vi "camara 2.1.vi"() -> ()   [LabVIEW 2010]
uses:
  <vilib>/addons/PixeLINK/Low Level Functions/CAMERA_FEATURES.llb/TDPU-CameraFeatures-FeatureIds.ctl
  <vilib>/addons/PixeLINK/Low Level Functions/CAMERA_FEATURES.llb/TDPU-CameraFeatures-FeatureFlags.ctl
  <vilib>/addons/PixeLINK/Low Level Functions/ACQUISITION.llb/TDPU-Acquisition-StreamState.ctl
  <vilib>/sound2/lvsound2.llb/Sampling Mode.ctl
  <vilib>/vision/NI_Vision_Development_Module.lvlib
  <vilib>/addons/PixeLINK/Low Level Functions/CAMERA_FEATURES.llb/TDPU-CameraFeatures-PixelFormat.ctl
  <vilib>/sound2/lvsound2.llb/Sound Data Format.ctl
panel:
  in  "SigmaMax (ms)":dbl
  in  "lamda (nm)":dbl
  in  "m":dbl
  in  "b":dbl
  in  "opticalPathMax (nm)":dbl
  out "contraste":u8
  in  "Sonido":bool
  in  "lamda (nm)":dbl
  in  "Frecuencia":dbl
  in  "sound format":T1={"sample rate (S/s)"=22050.0, "number of channels"=2, "bits per sample"=16}
  in  "Mostrar":bool
  in  "Blue":sgl(slide) scale=0.0..4.0
  in  "Green":sgl(slide) scale=0.0..4.0
  in  "Red":sgl(slide) scale=0.0..4.0
  in  "Gain":dbl(slide) scale=0.0..25.0
  out "Image":T2(plugin-control)
  in  "Exposure Time (ms)":dbl(slide) scale=0.1..2000.0
  in  "Streeam":bool
  in  "Pixel Format Requerido":T3 items=["PIXEL_FORMAT_MONO8", "PIXEL_FORMAT_MONO16", "PIXEL_FORMAT_YUV422", "PIXEL_FORMAT_BAYER8_GRBG", "PIXEL_FORMAT_BAYER16_GRBG", "PIXEL_FORMAT_RGB24", "PIXEL_FORMAT_RGB48", "PIXEL_FORMAT_BAYER8_RGGB", "PIXEL_FORMAT_BAYER8_GBRG ", "PIXEL_FORMAT_BAYER8_BGGR ", "PIXEL_FORMAT_BAYER16_RGGB ", "PIXEL_FORMAT_BAYER16_GBRG", "PIXEL_FORMAT_BAYER16_BGGR", "PIXEL_FORMAT_RGB32"]
  in  "Stop App":bool
  out "Numero de Camaras":u32
  in  "Selector":u16(ring) items=["776002034"]
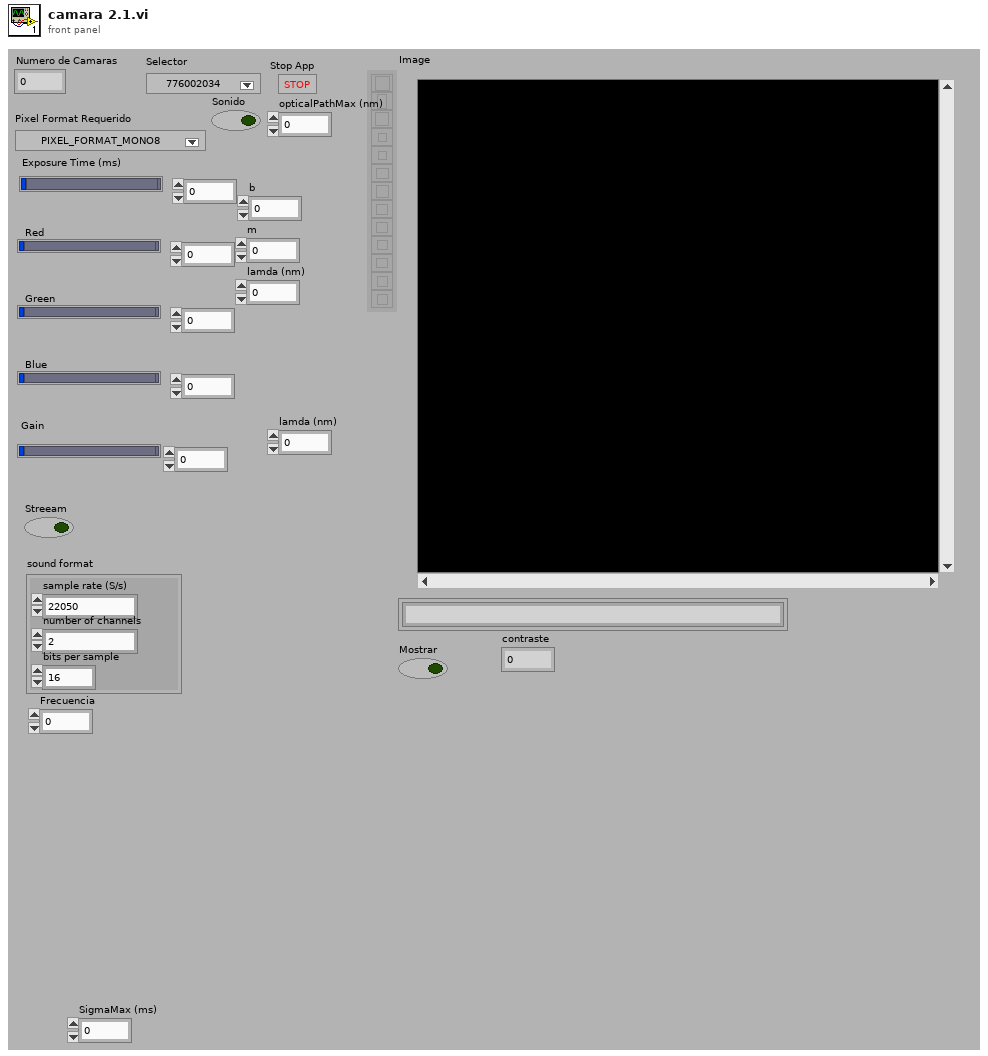
[diagram p1: front panel]
types:
  T1 = typedef "Sound Data Format.ctl" = cluster{"sample rate (S/s)":dbl, "number of channels":i32, "bits per sample":i32}
  T2 = typedef "IMAQ Image.ctl" = refnum<image>
  T3 = typedef "TDPU-CameraFeatures-PixelFormat.ctl" = u16
  T4 = typedef "Sampling Mode.ctl" = i32
  T5 = typedef "Image Type" = u32
  T6 = cluster{"sample rate (S/s)":dbl, "number of channels":i32, "bits per sample":i32}
  T7 = typedef "Sound Output Task ID.ctl" = u32
  T8 = cluster{"Red (or Hue) value":u8, "Green (or Sat) value":u8, "Blue (or Light or Val) value":u8}[]
  T9 = typedef "TDPU-Acquisition-StreamState.ctl" = u32
  T10 = typedef "TDPU-CameraFeatures-FeatureIds.ctl" = u32
  T11 = typedef "TDPU-CameraFeatures-FeatureFlags.ctl" = u32
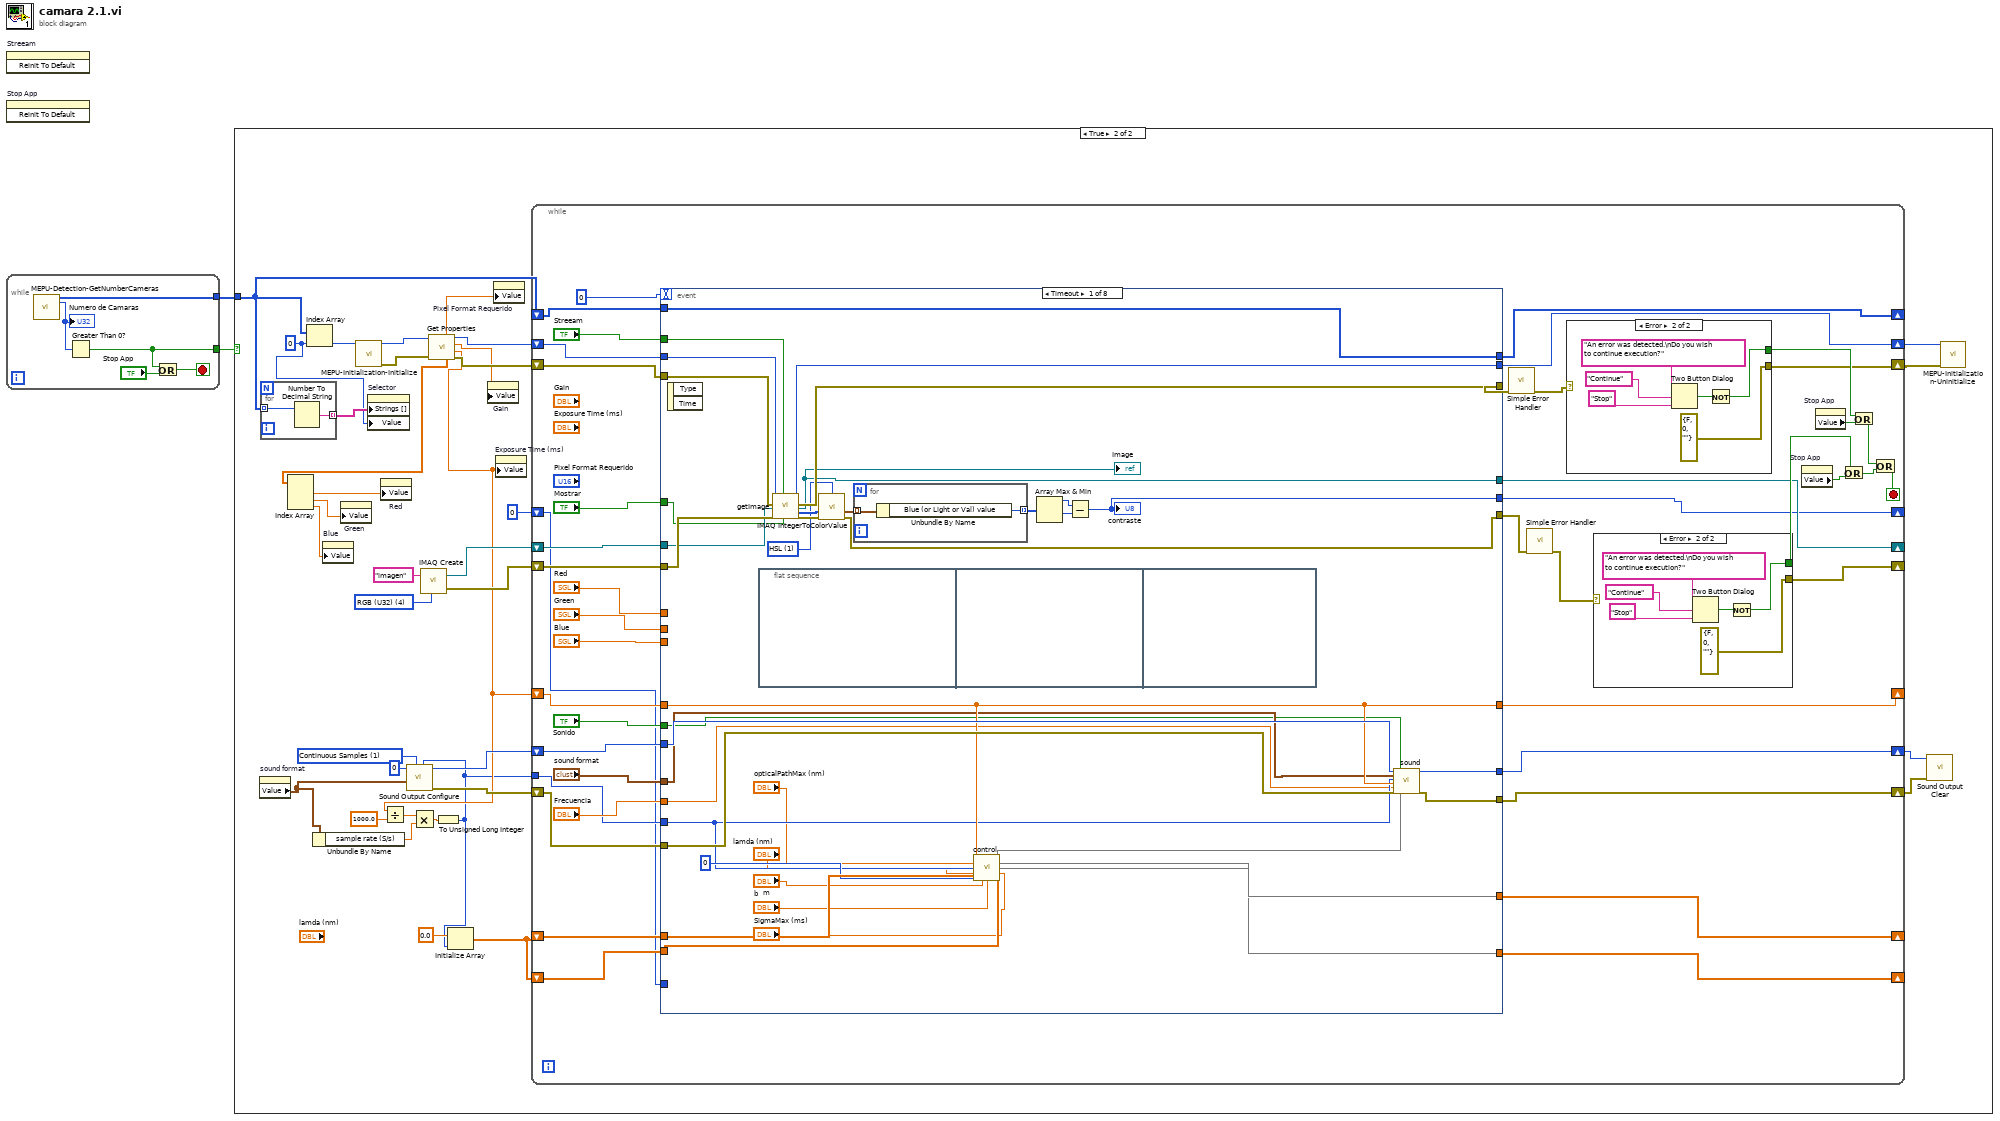
[diagram p0: block diagram]
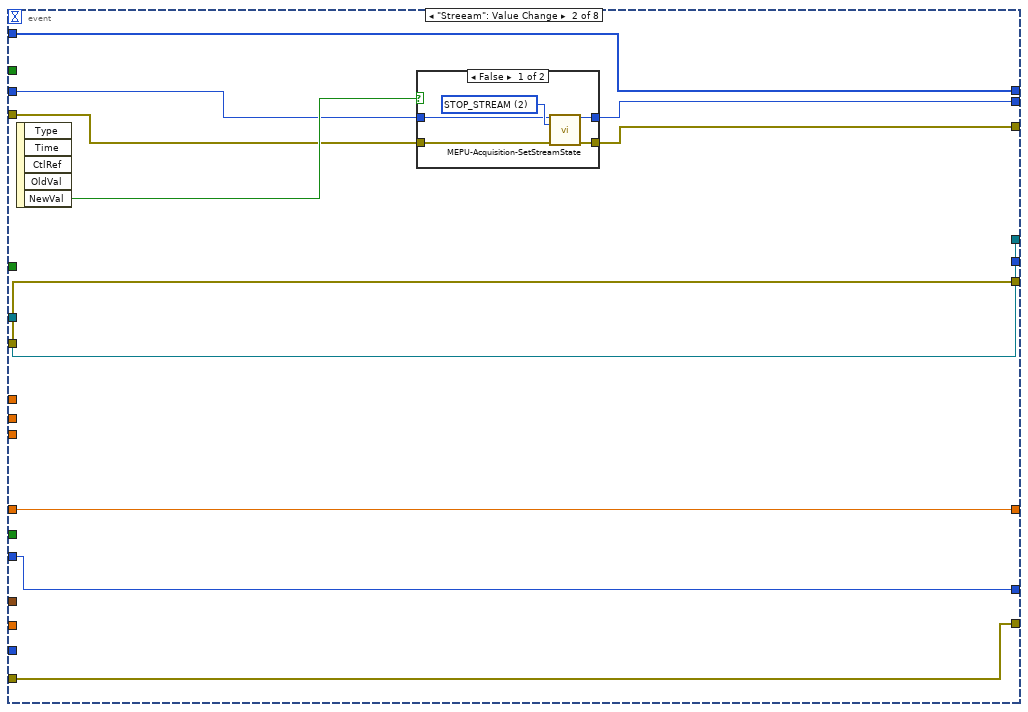
[diagram p5: hidden frame]
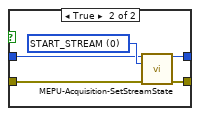
[diagram p6: hidden frame]
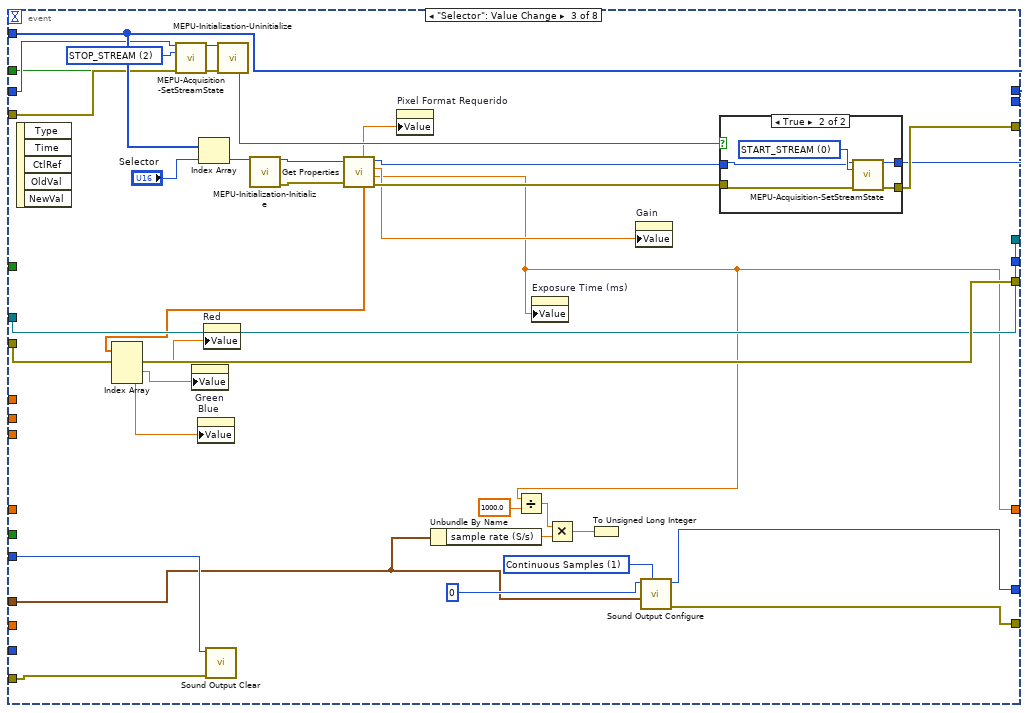
[diagram p7: hidden frame]
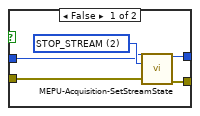
[diagram p8: hidden frame]
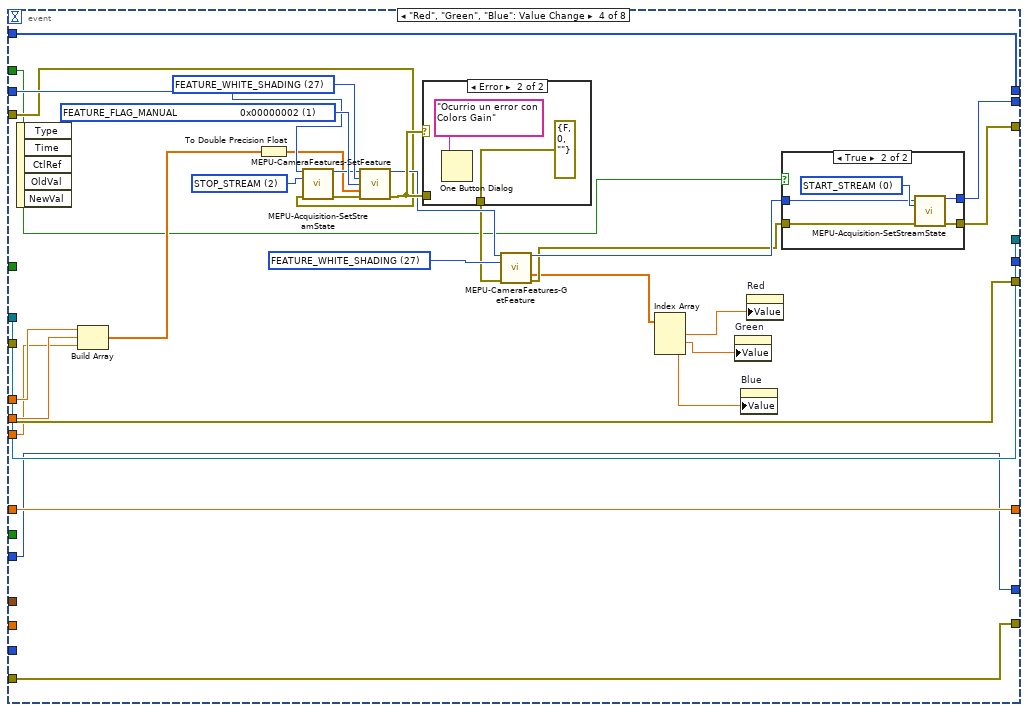
[diagram p9: hidden frame]
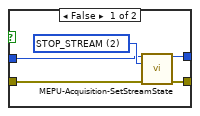
[diagram p10: hidden frame]
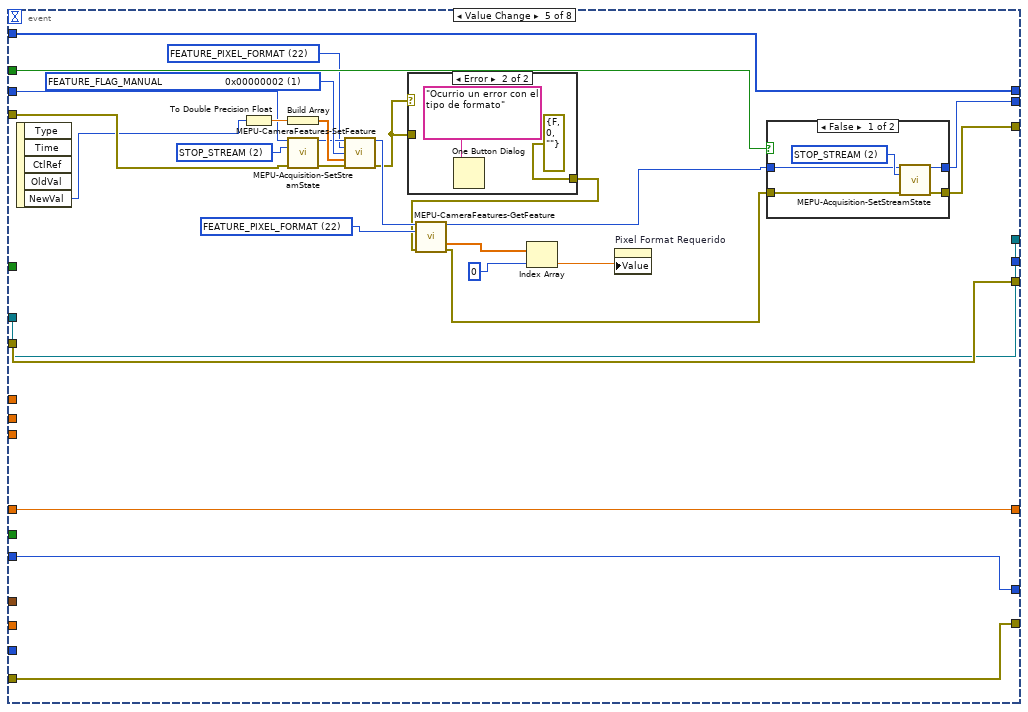
[diagram p12: hidden frame]
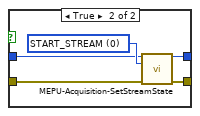
[diagram p13: hidden frame]
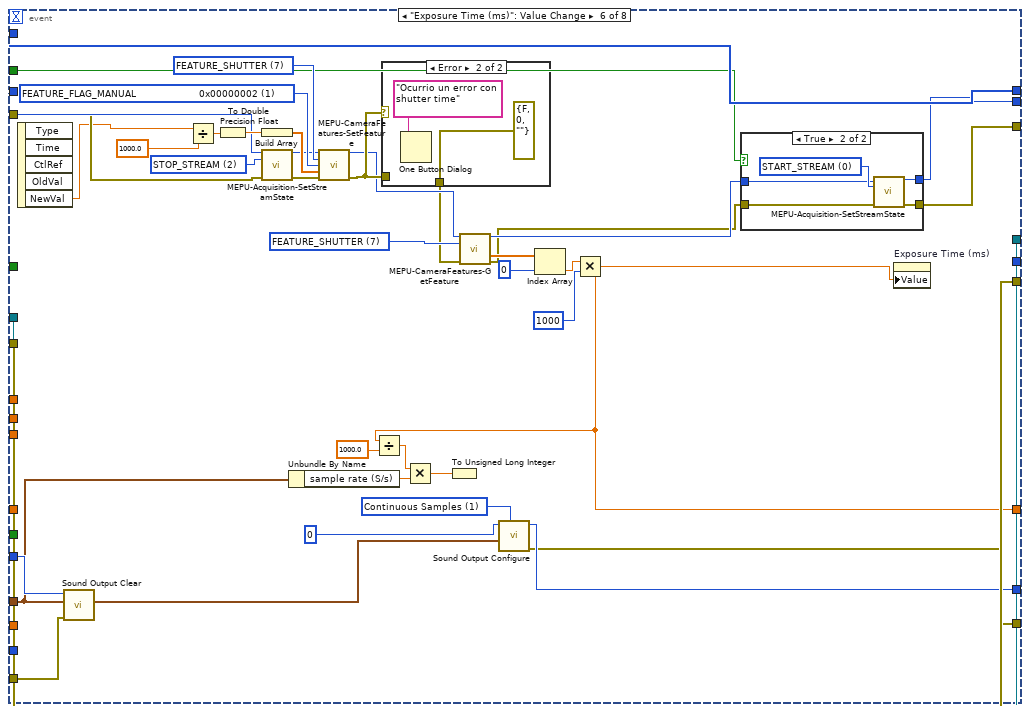
[diagram p15: hidden frame]
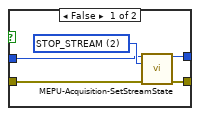
[diagram p16: hidden frame]
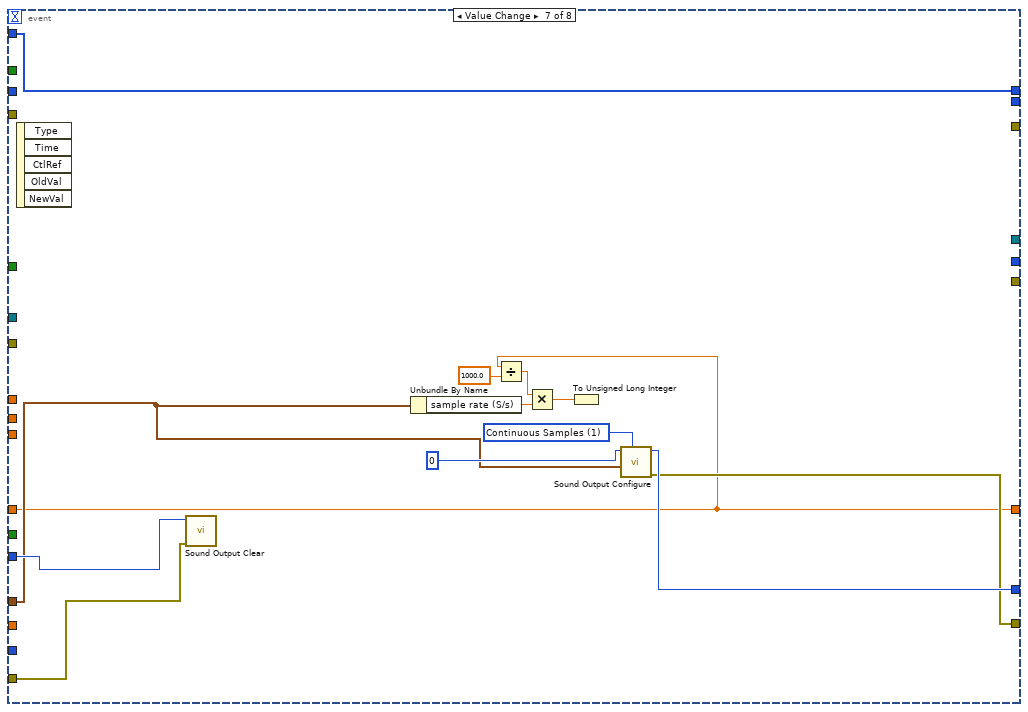
[diagram p18: hidden frame]
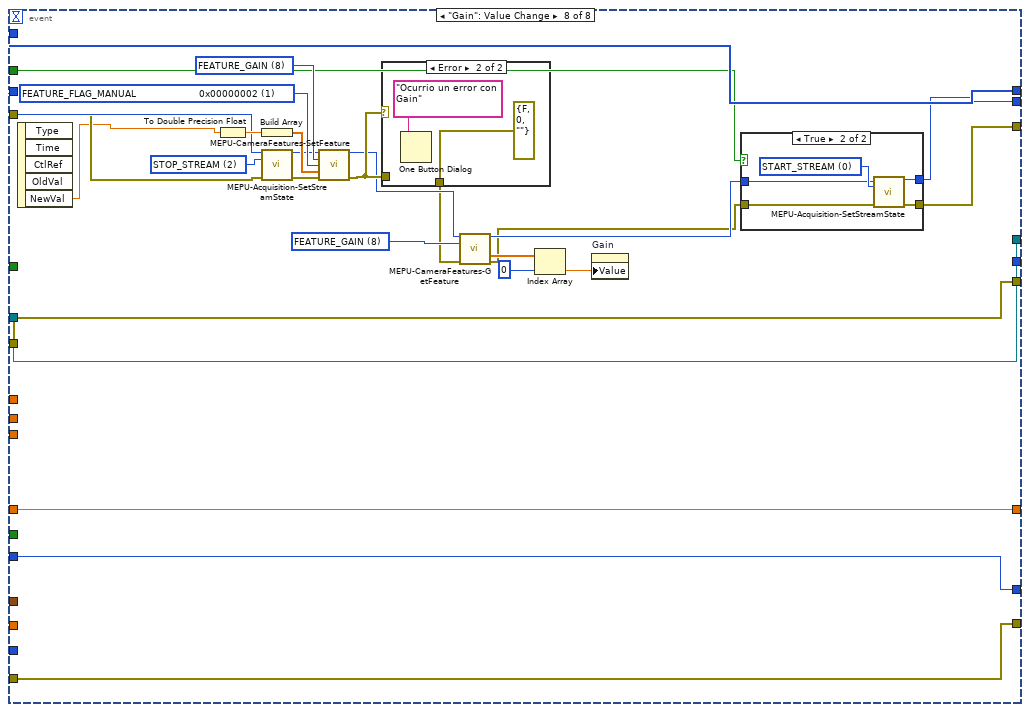
[diagram p19: hidden frame]
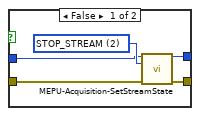
[diagram p20: hidden frame]
diagram:
  n1 = invoke on="Streeam" class="Bool (strict)" method="Reinit To Default"() -> ()  [unwired: 3 in, 3 out]
  n2 = invoke on="Stop App" class="Bool (strict)" method="Reinit To Default"() -> ()  [unwired: 3 in, 3 out]
  n3 = while {
    tunnel: [w7] -> w2
    tunnel: [w3] -> w1
    stop <- w5 stop-if-true
    n4 = call <vilib>:"MEPU-Detection-GetNumberCameras.vi"() -> ("LV_SerialNumbers OUT"=w7:u32[], "LV_NumberSerial OUT"=w4:u32)  [unwired: 13 in, 1 out]
    "Numero de Camaras" <- w4
    n5 = Greater Than 0?(x=w4) -> (x > 0?=w3:bool)
    n6 = Or(x=w3, y="Stop App") -> (x .or. y?=w5:bool)
  }
  n7 = case shown="True" w1 {
    tunnel: w2 -> [_ w41]
    frame False {
    }
    frame True {
      w24 = T4 1 items=["Finite Samples", "Continuous Samples"] ("sample mode")
      w35 = T5 4 items=["Grayscale (U8)", "Grayscale (I16)", "Grayscale (SGL)", "Complex (CSG)", "RGB (U32)", "HSL (U32)", "RGB (U64)", "Grayscale (U16)"] ("Image Type")
      w40 = 0
      n8 = property on="sound format" class="Clust (strict)"() -> ("Value"=w16:T6)  [unwired: 2 in, 2 out]
      n9 = for {
        tunnel: w41 -> [w403] mode=indexing
        tunnel: [w402] -> w43 mode=indexing
        n10 = Number To Decimal String(number=w403) -> (decimal integer string=w402:string)  [unwired: 1 in]
      }
      n11 = Index Array(array=w41, index=w40) -> (element=w42:u32)
      n12 = Unbundle By Name(w16) -> ("sample rate (S/s)"=w20:dbl)
      n13 = call <vilib>:"MEPU-Initialization-Initialize.vi"("uSerialNumber IN"=w42) -> ("phCamera OUT"=w34:u32, "Error OUT"=w33:errorcluster)  [unwired: 12 in, 1 out]
      n14 = property on="Selector" class="Ring (strict)"("Strings []"=w43, "Value"=w40) -> ()  [unwired: 2 in, 2 out]
      n15 = call "IMAQ Create"("Image Name"="imagen", "Image Type"=w35) -> ("New Image"=w38:T2, "error out"=w36:errorcluster)  [unwired: 3 in]
      n16 = call "Get Properties.vi"("hCamera IN"=w34, "Error IN"=w33) -> ("Pixel Format OUT"=w30:dbl, "hCamera OUT"=w32:u32, "Gain OUT"=w29:dbl, "Colors Gain OUT"=w25:dbl[], "Shutter Time OUT (ms)"=w15:dbl, "Error OUT"=w31:errorcluster)  [unwired: 3 in]
      n17 = Index Array(array=w25) -> (element #1=w28:dbl, element #2=w27:dbl, element #3=w26:dbl)  [unwired: 3 in]
      n18 = property on="Blue" class="Slide (strict)"("Value"=w26) -> ()  [unwired: 2 in, 2 out]
      n19 = property on="Green" class="Slide (strict)"("Value"=w27) -> ()  [unwired: 2 in, 2 out]
      n20 = property on="Red" class="Slide (strict)"("Value"=w28) -> ()  [unwired: 2 in, 2 out]
      n21 = Divide(x=w15, y=sgl 1000.0) -> (x/y=w19:dbl)
      n22 = Multiply(x=w19, y=w20) -> (x*y=w18:dbl)
      n23 = To Unsigned Long Integer(number=w18) -> (unsigned 32bit integer=w10:u32)
      n24 = call <vilib>:"Sound Output Configure.vi"("number of samples/ch"=w10, "sample mode"=w24, "sound format"=w16, "device ID"=u32 0) -> ("error out"=w21:errorcluster, "task ID"=w22:T7)  [unwired: 6 in]
      n25 = Initialize Array(0.0 ("element"), w10) -> (w9:dbl[])
      n26 = property on="Gain" class="Slide (strict)"("Value"=w29) -> ()  [unwired: 2 in, 2 out]
      n27 = property on="Pixel Format Requerido" class="Ring (strict)"("Value"=w30) -> ()  [unwired: 2 in, 2 out]
      n28 = property on="Exposure Time (ms)" class="Slide (strict)"("Value"=w15) -> ()  [unwired: 2 in, 2 out]
      n29 = while {
        shift-right: [w85] -> _
        shift-left: w41 -> [w86]
        shift-right: [w76] -> w39
        shift-left: w32 -> [w84]
        shift-right: [w80] -> w14
        shift-left: w31 -> [w83]
        shift-right: [w66] -> _
        shift-left: w36 -> [w65]
        shift-right: [w64] -> _
        shift-left: w38 -> [w74]
        shift-right: [w56] -> w13
        shift-left: w22 -> [w59]
        shift-right: [w55] -> w12
        shift-left: w21 -> [w58]
        shift-right: [w54] -> _
        shift-left: w15 -> [w53]
        shift-right: [w46] -> _
        shift-left: w9 -> [w50]
        shift-right: [w49] -> _
        shift-left: w9 -> [w48]
        tunnel: w10 -> [w47]
        shift-right: [w45] -> _
        shift-left: u8 0 -> [w44]
        stop <- w68 stop-if-true
        n30 = event shown="[0] Timeout" {
          selector: _ -> [_ _ _ _ _ _ _ _]
          dyn-events: _ -> [_ _ _ _ _ _ _ _]
          timeout: 0 -> [_ _ _ _ _ _ _ _]
          tunnel: w86 -> [w141 w147 w197 w240 w273 w326 w360 w380]
          tunnel: [w138 w151 w190 w224 w272 w325 _ w379] -> w76
          tunnel: [w137 w150 w191 w223 w271 w324 _ w378] -> w77
          tunnel: [w141 w147 w197 w240 w273 w326 w360 w380] -> w85
          tunnel: w84 -> [w140 w153 w192 w226 w278 w323 _ w377]
          tunnel: w83 -> [w139 w152 w193 w225 w277 w322 _ w376]
          tunnel: "Streeam" -> [w134 _ w189 w213 w270 w321 _ w375]
          tunnel: w74 -> [w135 w148 w187 w228 w258 w307 _ w366]
          tunnel: w65 -> [w136 w149 w188 w227 w269 w318 _ w374]
          tunnel: [w128 w149 w188 w227 w269 w318 _ w374] -> w73
          tunnel: [w133 w148 w187 w228 w258 w307 _ w366] -> w64
          tunnel: "Red" -> [_ _ _ w218 _ _ _ _]
          tunnel: "Green" -> [_ _ _ w217 _ _ _ _]
          tunnel: "Blue" -> [_ _ _ w216 _ _ _ _]
          tunnel: "Mostrar" -> [w132 _ _ _ _ _ _ _]
          tunnel: w59 -> [w118 w145 w170 w211 w255 w306 w353 w362]
          tunnel: w58 -> [w119 w144 w169 w210 w254 w305 w352 w361]
          tunnel: "sound format" -> [w114 _ w165 _ _ w298 w351 _]
          tunnel: [w112 w145 w168 w211 w255 w297 w350 w362] -> w56
          tunnel: [w111 w144 w167 w210 w254 w296 w349 w361] -> w55
          tunnel: w53 -> [w117 w146 _ w212 w256 _ w348 w363]
          tunnel: [w117 w146 w166 w212 w256 w295 w348 w363] -> w54
          tunnel: "Frecuencia" -> [w115 _ _ _ _ _ _ _]
          tunnel: "Sonido" -> [w113 _ _ _ _ _ _ _]
          tunnel: w50 -> [w123 _ _ _ _ _ _ _]
          tunnel: [w122 _ _ _ _ _ _ _] -> w49
          tunnel: w48 -> [w121 _ _ _ _ _ _ _]
          tunnel: w47 -> [w116 _ _ _ _ _ _ _]
          tunnel: [w110 _ _ _ _ _ _ _] -> w46
          tunnel: [w108 _ _ _ _ _ _ _] -> w45
          tunnel: w44 -> [_ _ _ _ _ _ _ _]
          event Timeout {
            w129 = u16 1 items=["RGB", "HSL", "HSV", "HSI"] ("Color Mode")
            n31 = event-data() -> ()  [unwired: 1 in, 2 out]
            n32 = flat-sequence {
              frame #0 {
              }
              frame #1 {
              }
              frame #2 {
              }
            }
            n33 = call "getImage.vi"("hCamera IN"=w140, "errorCamera IN"=w139, "Image IN"=w135, "imageError IN"=w136, "Streeam"=w134, "Show"=w132) -> ("hCamera OUT"=w138:u32, "errorCamera OUT"=w137:errorcluster, "Image OUT"=w133:T2, "1D RGB32 Array OUT"=w131:u32[], "errorImage OUT"=w130:errorcluster)  [unwired: 8 in, 1 out]
            "Image" <- w133
            n34 = call "IMAQ IntegerToColorValue"("error in (no error)"=w130, "1D U32 array"=w131, "Color Mode"=w129) -> ("1D Color value array"=w127:T8, "error out"=w128:errorcluster)  [unwired: 2 in, 2 out]
            n35 = for {
              tunnel: w127 -> [w143] mode=indexing
              tunnel: [w142] -> w126 mode=indexing
              n36 = Unbundle By Name(w143) -> ("Blue (or Light or Val) value"=w142:u8)
            }
            n37 = call "control.vi"("tiempo (ms)"=w117, "opticalPathMax (nm)"="opticalPathMax (nm)", "#samples"=w116, "lamda (nm)"="lamda (nm)", "SigmaMax (ms)"="SigmaMax (ms)", 11:0, "m"="m", "b"="b", 14:w121, 15:w123) -> (4:w109, 6:w122, 8:w110)  [unwired: 3 in]
            n38 = Array Max & Min(array=w126) -> (max value=w125:u8, min value=w124:u8)  [unwired: 2 out]
            n39 = Subtract(x=w125, y=w124) -> (x-y=w108:u8)
            "contraste" <- w108
            n40 = call "sound.vi"("task ID IN"=w118, "sound format"=w114, "# samples"=w116, "time (ms)"=w117, "Base frecuency"=w115, "error IN"=w119, "sound?"=w113, "df Array"=w109) -> ("task ID OUT"=w112:T7, "error OUT"=w111:errorcluster)  [unwired: 10 in]
          }
          event "Streeam": Value Change {
            n41 = event-data() -> ("NewVal"=w154:bool)  [unwired: 1 in, 4 out]
            n42 = case shown="False" w154 {
              tunnel: w153 -> [w158 w163]
              tunnel: w152 -> [w157 w162]
              tunnel: [w155 w161] -> w150
              tunnel: [w156 w160] -> w151
              frame False {
                w159 = T9 2 items=["START_STREAM", "PAUSE_STREAM", "STOP_STREAM"] ("uStreamState IN")
                n43 = call <vilib>:"MEPU-Acquisition-SetStreamState.vi"("hCamera IN"=w158, "uStreamState IN"=w159, "Error IN"=w157) -> ("hCamera OUT"=w156:u32, "Error OUT"=w155:errorcluster)  [unwired: 11 in]
              }
              frame True {
                w164 = T9 0 items=["START_STREAM", "PAUSE_STREAM", "STOP_STREAM"] ("uStreamState IN")
                n44 = call <vilib>:"MEPU-Acquisition-SetStreamState.vi"("hCamera IN"=w163, "uStreamState IN"=w164, "Error IN"=w162) -> ("hCamera OUT"=w160:u32, "Error OUT"=w161:errorcluster)  [unwired: 11 in]
              }
            }
          }
          event "Selector": Value Change {
            w176 = T4 1 items=["Finite Samples", "Continuous Samples"] ("sample mode")
            w196 = T9 2 items=["START_STREAM", "PAUSE_STREAM", "STOP_STREAM"] ("uStreamState IN")
            n45 = event-data() -> ()  [unwired: 1 in, 5 out]
            n46 = call <vilib>:"MEPU-Acquisition-SetStreamState.vi"("hCamera IN"=w192, "uStreamState IN"=w196, "Error IN"=w193) -> ("hCamera OUT"=w194:u32, "Error OUT"=w195:errorcluster)  [unwired: 11 in]
            n47 = Index Array(array=w197, index="Selector") -> (element=w198:u32)
            n48 = call <vilib>:"Sound Output Clear.vi"("error in (no error)"=w169, "task ID"=w170) -> ()  [unwired: 9 in, 1 out]
            n49 = call <vilib>:"MEPU-Initialization-Uninitialize.vi"("hCamera IN"=w194, "Error IN"=w195) -> ()  [unwired: 13 in, 1 out]
            n50 = call <vilib>:"MEPU-Initialization-Initialize.vi"("uSerialNumber IN"=w198) -> ("phCamera OUT"=w183:u32, "Error OUT"=w182:errorcluster)  [unwired: 12 in, 1 out]
            n51 = call "Get Properties.vi"("hCamera IN"=w183, "Error IN"=w182) -> ("Pixel Format OUT"=w181:dbl, "hCamera OUT"=w179:u32, "Gain OUT"=w178:dbl, "Colors Gain OUT"=w177:dbl[], "Shutter Time OUT (ms)"=w166:dbl, "Error OUT"=w180:errorcluster)  [unwired: 3 in]
            n52 = Index Array(array=w177) -> (element #1=w186:dbl, element #2=w185:dbl, element #3=w184:dbl)  [unwired: 3 in]
            n53 = property on="Green" class="Slide (strict)"("Value"=w185) -> ()  [unwired: 2 in, 2 out]
            n54 = property on="Blue" class="Slide (strict)"("Value"=w184) -> ()  [unwired: 2 in, 2 out]
            n55 = property on="Red" class="Slide (strict)"("Value"=w186) -> ()  [unwired: 2 in, 2 out]
            n56 = property on="Pixel Format Requerido" class="Ring (strict)"("Value"=w181) -> ()  [unwired: 2 in, 2 out]
            n57 = Unbundle By Name(w165) -> ("sample rate (S/s)"=w174:dbl)
            n58 = Divide(x=w166, y=sgl 1000.0) -> (x/y=w173:dbl)
            n59 = property on="Exposure Time (ms)" class="Slide (strict)"("Value"=w166) -> ()  [unwired: 2 in, 2 out]
            n60 = Multiply(x=w173, y=w174) -> (x*y=w172:dbl)
            n61 = To Unsigned Long Integer(number=w172) -> ()  [unwired: 1 out]
            n62 = property on="Gain" class="Slide (strict)"("Value"=w178) -> ()  [unwired: 2 in, 2 out]
            n63 = call <vilib>:"Sound Output Configure.vi"("sample mode"=w176, "sound format"=w165, "device ID"=u32 0) -> ("error out"=w167:errorcluster, "task ID"=w168:T7)  [unwired: 7 in]
            n64 = case shown="True" w189 {
              tunnel: [w202 w208] -> w191
              tunnel: [w203 w207] -> w190
              tunnel: w180 -> [w201 w206]
              tunnel: w179 -> [w200 w205]
              frame False {
                w204 = T9 2 items=["START_STREAM", "PAUSE_STREAM", "STOP_STREAM"] ("uStreamState IN")
                n65 = call <vilib>:"MEPU-Acquisition-SetStreamState.vi"("hCamera IN"=w200, "uStreamState IN"=w204, "Error IN"=w201) -> ("hCamera OUT"=w203:u32, "Error OUT"=w202:errorcluster)  [unwired: 11 in]
              }
              frame True {
                w209 = T9 0 items=["START_STREAM", "PAUSE_STREAM", "STOP_STREAM"] ("uStreamState IN")
                n66 = call <vilib>:"MEPU-Acquisition-SetStreamState.vi"("hCamera IN"=w205, "uStreamState IN"=w209, "Error IN"=w206) -> ("hCamera OUT"=w207:u32, "Error OUT"=w208:errorcluster)  [unwired: 11 in]
              }
            }
          }
          event "Red", "Green", "Blue": Value Change {
            w233 = T10 27 items=["FEATURE_BRIGHTNESS", "FEATURE_EXPOSURE", "FEATURE_SHARPNESS", "FEATURE_WHITE_BAL", "FEATURE_HUE", "FEATURE_SATURATION", "FEATURE_GAMMA", "FEATURE_SHUTTER", "FEATURE_GAIN", "FEATURE_IRIS", "FEATURE_FOCUS", "FEATURE_TEMPERATURE", "FEATURE_TRIGGER", "FEATURE_ZOOM", "FEATURE_PAN", "FEATURE_TILT", "FEATURE_OPT_FILTER", "FEATURE_GPIO", "FEATURE_FRAME_RATE", "FEATURE_ROI", "FEATURE_FLIP", "FEATURE_PIXEL_ADDRESSING", "FEATURE_PIXEL_FORMAT", "FEATURE_EXTENDED_SHUTTER", "FEATURE_AUTO_ROI", "FEATURE_LOOKUP_TABLE", "FEATURE_MEMORY_CHANNEL", "FEATURE_WHITE_SHADING", "FEATURE_ROTATE", "FEATURE_IMAGER_CLK_DIVISOR", "FEATURE_TRIG_WITH_CNTRLD_LIGHT", "FEATURE_MAX_PIXEL_SIZE"] ("uFeatureId IN")
            w234 = T9 2 items=["START_STREAM", "PAUSE_STREAM", "STOP_STREAM"] ("uStreamState IN")
            w238 = T11 1 items=["FEATURE_FLAG_PRESENCE                 0x00000001", "FEATURE_FLAG_MANUAL                     0x00000002", "FEATURE_FLAG_AUTO                         0x00000004", "FEATURE_FLAG_ONEPUSH                   0x00000008", "FEATURE_FLAG_OFF                            0x00000010", "FEATURE_FLAG_DESC_SUPPORTED    0x00000020", "FEATURE_FLAG_READ_ONLY               0x00000040"] ("uFlags IN")
            w239 = T10 27 items=["FEATURE_BRIGHTNESS", "FEATURE_EXPOSURE", "FEATURE_SHARPNESS", "FEATURE_WHITE_BAL", "FEATURE_HUE", "FEATURE_SATURATION", "FEATURE_GAMMA", "FEATURE_SHUTTER", "FEATURE_GAIN", "FEATURE_IRIS", "FEATURE_FOCUS", "FEATURE_TEMPERATURE", "FEATURE_TRIGGER", "FEATURE_ZOOM", "FEATURE_PAN", "FEATURE_TILT", "FEATURE_OPT_FILTER", "FEATURE_GPIO", "FEATURE_FRAME_RATE", "FEATURE_ROI", "FEATURE_FLIP", "FEATURE_PIXEL_ADDRESSING", "FEATURE_PIXEL_FORMAT", "FEATURE_EXTENDED_SHUTTER", "FEATURE_AUTO_ROI", "FEATURE_LOOKUP_TABLE", "FEATURE_MEMORY_CHANNEL", "FEATURE_WHITE_SHADING", "FEATURE_ROTATE", "FEATURE_IMAGER_CLK_DIVISOR", "FEATURE_TRIG_WITH_CNTRLD_LIGHT", "FEATURE_MAX_PIXEL_SIZE"] ("uFeatureId IN")
            n67 = event-data() -> ()  [unwired: 1 in, 5 out]
            n68 = Build Array(w218, w217, w216) -> (w215:sgl[])
            n69 = To Double Precision Float(number=w215) -> (double precision float=w214:dbl[])
            n70 = call <vilib>:"MEPU-Acquisition-SetStreamState.vi"("hCamera IN"=w226, "uStreamState IN"=w234, "Error IN"=w225) -> ("hCamera OUT"=w236:u32, "Error OUT"=w235:errorcluster)  [unwired: 11 in]
            n71 = call <vilib>:"MEPU-CameraFeatures-SetFeature.vi"("hCamera IN"=w236, "uFeatureId IN"=w239, "uFlags IN"=w238, "pParms IN"=w214, "Error IN"=w235) -> ("hCamera OUT"=w232:u32, "Error OUT"=w237:errorcluster)  [unwired: 8 in, 1 out]
            n72 = case shown="Error" w237 {
              tunnel: [w251 errorcluster {"status"=FALSE, "code"=0, "source"=""} ("Error OUT")] -> w229
              tunnel: w237 -> [w251 _]
              frame No Error {
              }
              frame Error {
                n73 = One Button Dialog(message="Ocurrio un error con Colors Gain") -> ()  [unwired: 1 in, 1 out]
              }
            }
            n74 = call <vilib>:"MEPU-CameraFeatures-GetFeature.vi"("hCamera IN"=w232, "uFeatureId IN"=w233, "Error IN"=w229) -> ("hCamera OUT"=w231:u32, "pParms OUT"=w219:dbl[], "Error OUT"=w230:errorcluster)  [unwired: 8 in, 2 out]
            n75 = Index Array(array=w219) -> (element #1=w222:dbl, element #2=w221:dbl, element #3=w220:dbl)  [unwired: 3 in]
            n76 = property on="Green" class="Slide (strict)"("Value"=w221) -> ()  [unwired: 2 in, 2 out]
            n77 = property on="Blue" class="Slide (strict)"("Value"=w220) -> ()  [unwired: 2 in, 2 out]
            n78 = property on="Red" class="Slide (strict)"("Value"=w222) -> ()  [unwired: 2 in, 2 out]
            n79 = case shown="True" w213 {
              tunnel: w230 -> [w244 w249]
              tunnel: [w242 w248] -> w223
              tunnel: [w243 w247] -> w224
              tunnel: w231 -> [w241 w246]
              frame False {
                w245 = T9 2 items=["START_STREAM", "PAUSE_STREAM", "STOP_STREAM"] ("uStreamState IN")
                n80 = call <vilib>:"MEPU-Acquisition-SetStreamState.vi"("hCamera IN"=w241, "uStreamState IN"=w245, "Error IN"=w244) -> ("hCamera OUT"=w243:u32, "Error OUT"=w242:errorcluster)  [unwired: 11 in]
              }
              frame True {
                w250 = T9 0 items=["START_STREAM", "PAUSE_STREAM", "STOP_STREAM"] ("uStreamState IN")
                n81 = call <vilib>:"MEPU-Acquisition-SetStreamState.vi"("hCamera IN"=w246, "uStreamState IN"=w250, "Error IN"=w249) -> ("hCamera OUT"=w247:u32, "Error OUT"=w248:errorcluster)  [unwired: 11 in]
              }
            }
          }
          event Value Change {
            w263 = T10 22 items=["FEATURE_BRIGHTNESS", "FEATURE_EXPOSURE", "FEATURE_SHARPNESS", "FEATURE_WHITE_BAL", "FEATURE_HUE", "FEATURE_SATURATION", "FEATURE_GAMMA", "FEATURE_SHUTTER", "FEATURE_GAIN", "FEATURE_IRIS", "FEATURE_FOCUS", "FEATURE_TEMPERATURE", "FEATURE_TRIGGER", "FEATURE_ZOOM", "FEATURE_PAN", "FEATURE_TILT", "FEATURE_OPT_FILTER", "FEATURE_GPIO", "FEATURE_FRAME_RATE", "FEATURE_ROI", "FEATURE_FLIP", "FEATURE_PIXEL_ADDRESSING", "FEATURE_PIXEL_FORMAT", "FEATURE_EXTENDED_SHUTTER", "FEATURE_AUTO_ROI", "FEATURE_LOOKUP_TABLE", "FEATURE_MEMORY_CHANNEL", "FEATURE_WHITE_SHADING", "FEATURE_ROTATE", "FEATURE_IMAGER_CLK_DIVISOR", "FEATURE_TRIG_WITH_CNTRLD_LIGHT", "FEATURE_MAX_PIXEL_SIZE"] ("uFeatureId IN")
            w274 = T9 2 items=["START_STREAM", "PAUSE_STREAM", "STOP_STREAM"] ("uStreamState IN")
            w281 = T11 1 items=["FEATURE_FLAG_PRESENCE                 0x00000001", "FEATURE_FLAG_MANUAL                     0x00000002", "FEATURE_FLAG_AUTO                         0x00000004", "FEATURE_FLAG_ONEPUSH                   0x00000008", "FEATURE_FLAG_OFF                            0x00000010", "FEATURE_FLAG_DESC_SUPPORTED    0x00000020", "FEATURE_FLAG_READ_ONLY               0x00000040"] ("uFlags IN")
            w268 = T10 22 items=["FEATURE_BRIGHTNESS", "FEATURE_EXPOSURE", "FEATURE_SHARPNESS", "FEATURE_WHITE_BAL", "FEATURE_HUE", "FEATURE_SATURATION", "FEATURE_GAMMA", "FEATURE_SHUTTER", "FEATURE_GAIN", "FEATURE_IRIS", "FEATURE_FOCUS", "FEATURE_TEMPERATURE", "FEATURE_TRIGGER", "FEATURE_ZOOM", "FEATURE_PAN", "FEATURE_TILT", "FEATURE_OPT_FILTER", "FEATURE_GPIO", "FEATURE_FRAME_RATE", "FEATURE_ROI", "FEATURE_FLIP", "FEATURE_PIXEL_ADDRESSING", "FEATURE_PIXEL_FORMAT", "FEATURE_EXTENDED_SHUTTER", "FEATURE_AUTO_ROI", "FEATURE_LOOKUP_TABLE", "FEATURE_MEMORY_CHANNEL", "FEATURE_WHITE_SHADING", "FEATURE_ROTATE", "FEATURE_IMAGER_CLK_DIVISOR", "FEATURE_TRIG_WITH_CNTRLD_LIGHT", "FEATURE_MAX_PIXEL_SIZE"] ("uFeatureId IN")
            n82 = event-data() -> ("NewVal"=w259:T3)  [unwired: 1 in, 4 out]
            n83 = To Double Precision Float(number=w259) -> (double precision float=w279:dbl)
            n84 = Build Array(w279) -> (w280:dbl[])
            n85 = call <vilib>:"MEPU-Acquisition-SetStreamState.vi"("hCamera IN"=w278, "uStreamState IN"=w274, "Error IN"=w277) -> ("hCamera OUT"=w276:u32, "Error OUT"=w275:errorcluster)  [unwired: 11 in]
            n86 = call <vilib>:"MEPU-CameraFeatures-SetFeature.vi"("hCamera IN"=w276, "uFeatureId IN"=w268, "uFlags IN"=w281, "pParms IN"=w280, "Error IN"=w275) -> ("hCamera OUT"=w265:u32, "Error OUT"=w261:errorcluster)  [unwired: 8 in, 1 out]
            n87 = case shown="Error" w261 {
              tunnel: [w292 errorcluster {"status"=FALSE, "code"=0, "source"=""} ("Error OUT")] -> w260
              tunnel: w261 -> [w292 _]
              frame No Error {
              }
              frame Error {
                n88 = One Button Dialog(message="Ocurrio un error con el tipo de formato") -> ()  [unwired: 1 in, 1 out]
              }
            }
            n89 = call <vilib>:"MEPU-CameraFeatures-GetFeature.vi"("hCamera IN"=w265, "uFeatureId IN"=w263, "Error IN"=w260) -> ("hCamera OUT"=w264:u32, "pParms OUT"=w262:dbl[], "Error OUT"=w266:errorcluster)  [unwired: 8 in, 2 out]
            n90 = Index Array(array=w262, index=0) -> (element=w257:dbl)
            n91 = property on="Pixel Format Requerido" class="Ring (strict)"("Value"=w257) -> ()  [unwired: 2 in, 2 out]
            n92 = case shown="False" w270 {
              tunnel: w264 -> [w285 w290]
              tunnel: w266 -> [w284 w289]
              tunnel: [w282 w288] -> w271
              tunnel: [w283 w287] -> w272
              frame False {
                w286 = T9 2 items=["START_STREAM", "PAUSE_STREAM", "STOP_STREAM"] ("uStreamState IN")
                n93 = call <vilib>:"MEPU-Acquisition-SetStreamState.vi"("hCamera IN"=w285, "uStreamState IN"=w286, "Error IN"=w284) -> ("hCamera OUT"=w283:u32, "Error OUT"=w282:errorcluster)  [unwired: 11 in]
              }
              frame True {
                w291 = T9 0 items=["START_STREAM", "PAUSE_STREAM", "STOP_STREAM"] ("uStreamState IN")
                n94 = call <vilib>:"MEPU-Acquisition-SetStreamState.vi"("hCamera IN"=w290, "uStreamState IN"=w291, "Error IN"=w289) -> ("hCamera OUT"=w287:u32, "Error OUT"=w288:errorcluster)  [unwired: 11 in]
              }
            }
          }
          event "Exposure Time (ms)": Value Change {
            w304 = T4 1 items=["Finite Samples", "Continuous Samples"] ("sample mode")
            w313 = T10 7 items=["FEATURE_BRIGHTNESS", "FEATURE_EXPOSURE", "FEATURE_SHARPNESS", "FEATURE_WHITE_BAL", "FEATURE_HUE", "FEATURE_SATURATION", "FEATURE_GAMMA", "FEATURE_SHUTTER", "FEATURE_GAIN", "FEATURE_IRIS", "FEATURE_FOCUS", "FEATURE_TEMPERATURE", "FEATURE_TRIGGER", "FEATURE_ZOOM", "FEATURE_PAN", "FEATURE_TILT", "FEATURE_OPT_FILTER", "FEATURE_GPIO", "FEATURE_FRAME_RATE", "FEATURE_ROI", "FEATURE_FLIP", "FEATURE_PIXEL_ADDRESSING", "FEATURE_PIXEL_FORMAT", "FEATURE_EXTENDED_SHUTTER", "FEATURE_AUTO_ROI", "FEATURE_LOOKUP_TABLE", "FEATURE_MEMORY_CHANNEL", "FEATURE_WHITE_SHADING", "FEATURE_ROTATE", "FEATURE_IMAGER_CLK_DIVISOR", "FEATURE_TRIG_WITH_CNTRLD_LIGHT", "FEATURE_MAX_PIXEL_SIZE"] ("uFeatureId IN")
            w327 = T9 2 items=["START_STREAM", "PAUSE_STREAM", "STOP_STREAM"] ("uStreamState IN")
            w333 = T11 1 items=["FEATURE_FLAG_PRESENCE                 0x00000001", "FEATURE_FLAG_MANUAL                     0x00000002", "FEATURE_FLAG_AUTO                         0x00000004", "FEATURE_FLAG_ONEPUSH                   0x00000008", "FEATURE_FLAG_OFF                            0x00000010", "FEATURE_FLAG_DESC_SUPPORTED    0x00000020", "FEATURE_FLAG_READ_ONLY               0x00000040"] ("uFlags IN")
            w334 = T10 7 items=["FEATURE_BRIGHTNESS", "FEATURE_EXPOSURE", "FEATURE_SHARPNESS", "FEATURE_WHITE_BAL", "FEATURE_HUE", "FEATURE_SATURATION", "FEATURE_GAMMA", "FEATURE_SHUTTER", "FEATURE_GAIN", "FEATURE_IRIS", "FEATURE_FOCUS", "FEATURE_TEMPERATURE", "FEATURE_TRIGGER", "FEATURE_ZOOM", "FEATURE_PAN", "FEATURE_TILT", "FEATURE_OPT_FILTER", "FEATURE_GPIO", "FEATURE_FRAME_RATE", "FEATURE_ROI", "FEATURE_FLIP", "FEATURE_PIXEL_ADDRESSING", "FEATURE_PIXEL_FORMAT", "FEATURE_EXTENDED_SHUTTER", "FEATURE_AUTO_ROI", "FEATURE_LOOKUP_TABLE", "FEATURE_MEMORY_CHANNEL", "FEATURE_WHITE_SHADING", "FEATURE_ROTATE", "FEATURE_IMAGER_CLK_DIVISOR", "FEATURE_TRIG_WITH_CNTRLD_LIGHT", "FEATURE_MAX_PIXEL_SIZE"] ("uFeatureId IN")
            n95 = event-data() -> ("NewVal"=w308:dbl)  [unwired: 1 in, 4 out]
            n96 = call <vilib>:"Sound Output Clear.vi"("error in (no error)"=w305, "task ID"=w306) -> ()  [unwired: 9 in, 1 out]
            n97 = Divide(x=w308, y=1000.0) -> (x/y=w320:dbl)
            n98 = To Double Precision Float(number=w320) -> (double precision float=w331:dbl)
            n99 = Build Array(w331) -> (w332:dbl[])
            n100 = call <vilib>:"MEPU-Acquisition-SetStreamState.vi"("hCamera IN"=w323, "uStreamState IN"=w327, "Error IN"=w322) -> ("hCamera OUT"=w329:u32, "Error OUT"=w328:errorcluster)  [unwired: 11 in]
            n101 = Unbundle By Name(w298) -> ("sample rate (S/s)"=w302:dbl)
            n102 = call <vilib>:"MEPU-CameraFeatures-SetFeature.vi"("hCamera IN"=w329, "uFeatureId IN"=w334, "uFlags IN"=w333, "pParms IN"=w332, "Error IN"=w328) -> ("hCamera OUT"=w312:u32, "Error OUT"=w330:errorcluster)  [unwired: 8 in, 1 out]
            n103 = case shown="Error" w330 {
              tunnel: [w345 errorcluster {"status"=FALSE, "code"=0, "source"=""} ("Error OUT")] -> w309
              tunnel: w330 -> [w345 _]
              frame No Error {
              }
              frame Error {
                n104 = One Button Dialog(message="Ocurrio un error con shutter time") -> ()  [unwired: 1 in, 1 out]
              }
            }
            n105 = call <vilib>:"MEPU-CameraFeatures-GetFeature.vi"("hCamera IN"=w312, "uFeatureId IN"=w313, "Error IN"=w309) -> ("hCamera OUT"=w311:u32, "pParms OUT"=w314:dbl[], "Error OUT"=w310:errorcluster)  [unwired: 8 in, 2 out]
            n106 = call <vilib>:"Sound Output Configure.vi"("sample mode"=w304, "sound format"=w298, "device ID"=u32 0) -> ("error out"=w296:errorcluster, "task ID"=w297:T7)  [unwired: 7 in]
            n107 = Index Array(array=w314, index=0) -> (element=w317:dbl)
            n108 = Multiply(x=w317, y=1000) -> (x*y=w295:dbl)
            n109 = Divide(x=w295, y=sgl 1000.0) -> (x/y=w301:dbl)
            n110 = Multiply(x=w301, y=w302) -> (x*y=w300:dbl)
            n111 = To Unsigned Long Integer(number=w300) -> ()  [unwired: 1 out]
            n112 = case shown="True" w321 {
              tunnel: w310 -> [w338 w343]
              tunnel: [w336 w342] -> w324
              tunnel: [w337 w341] -> w325
              tunnel: w311 -> [w335 w340]
              frame False {
                w339 = T9 2 items=["START_STREAM", "PAUSE_STREAM", "STOP_STREAM"] ("uStreamState IN")
                n113 = call <vilib>:"MEPU-Acquisition-SetStreamState.vi"("hCamera IN"=w335, "uStreamState IN"=w339, "Error IN"=w338) -> ("hCamera OUT"=w337:u32, "Error OUT"=w336:errorcluster)  [unwired: 11 in]
              }
              frame True {
                w344 = T9 0 items=["START_STREAM", "PAUSE_STREAM", "STOP_STREAM"] ("uStreamState IN")
                n114 = call <vilib>:"MEPU-Acquisition-SetStreamState.vi"("hCamera IN"=w340, "uStreamState IN"=w344, "Error IN"=w343) -> ("hCamera OUT"=w341:u32, "Error OUT"=w342:errorcluster)  [unwired: 11 in]
              }
            }
            n115 = property on="Exposure Time (ms)" class="Slide (strict)"("Value"=w295) -> ()  [unwired: 2 in, 2 out]
          }
          event Value Change {
            w359 = T4 1 items=["Finite Samples", "Continuous Samples"] ("sample mode")
            n116 = event-data() -> ()  [unwired: 1 in, 5 out]
            n117 = call <vilib>:"Sound Output Clear.vi"("error in (no error)"=w352, "task ID"=w353) -> ()  [unwired: 9 in, 1 out]
            n118 = Unbundle By Name(w351) -> ("sample rate (S/s)"=w357:dbl)
            n119 = Divide(x=w348, y=sgl 1000.0) -> (x/y=w356:dbl)
            n120 = Multiply(x=w356, y=w357) -> (x*y=w355:dbl)
            n121 = To Unsigned Long Integer(number=w355) -> ()  [unwired: 1 out]
            n122 = call <vilib>:"Sound Output Configure.vi"("sample mode"=w359, "sound format"=w351, "device ID"=u32 0) -> ("error out"=w349:errorcluster, "task ID"=w350:T7)  [unwired: 7 in]
          }
          event "Gain": Value Change {
            w371 = T10 8 items=["FEATURE_BRIGHTNESS", "FEATURE_EXPOSURE", "FEATURE_SHARPNESS", "FEATURE_WHITE_BAL", "FEATURE_HUE", "FEATURE_SATURATION", "FEATURE_GAMMA", "FEATURE_SHUTTER", "FEATURE_GAIN", "FEATURE_IRIS", "FEATURE_FOCUS", "FEATURE_TEMPERATURE", "FEATURE_TRIGGER", "FEATURE_ZOOM", "FEATURE_PAN", "FEATURE_TILT", "FEATURE_OPT_FILTER", "FEATURE_GPIO", "FEATURE_FRAME_RATE", "FEATURE_ROI", "FEATURE_FLIP", "FEATURE_PIXEL_ADDRESSING", "FEATURE_PIXEL_FORMAT", "FEATURE_EXTENDED_SHUTTER", "FEATURE_AUTO_ROI", "FEATURE_LOOKUP_TABLE", "FEATURE_MEMORY_CHANNEL", "FEATURE_WHITE_SHADING", "FEATURE_ROTATE", "FEATURE_IMAGER_CLK_DIVISOR", "FEATURE_TRIG_WITH_CNTRLD_LIGHT", "FEATURE_MAX_PIXEL_SIZE"] ("uFeatureId IN")
            w381 = T9 2 items=["START_STREAM", "PAUSE_STREAM", "STOP_STREAM"] ("uStreamState IN")
            w387 = T11 1 items=["FEATURE_FLAG_PRESENCE                 0x00000001", "FEATURE_FLAG_MANUAL                     0x00000002", "FEATURE_FLAG_AUTO                         0x00000004", "FEATURE_FLAG_ONEPUSH                   0x00000008", "FEATURE_FLAG_OFF                            0x00000010", "FEATURE_FLAG_DESC_SUPPORTED    0x00000020", "FEATURE_FLAG_READ_ONLY               0x00000040"] ("uFlags IN")
            w388 = T10 8 items=["FEATURE_BRIGHTNESS", "FEATURE_EXPOSURE", "FEATURE_SHARPNESS", "FEATURE_WHITE_BAL", "FEATURE_HUE", "FEATURE_SATURATION", "FEATURE_GAMMA", "FEATURE_SHUTTER", "FEATURE_GAIN", "FEATURE_IRIS", "FEATURE_FOCUS", "FEATURE_TEMPERATURE", "FEATURE_TRIGGER", "FEATURE_ZOOM", "FEATURE_PAN", "FEATURE_TILT", "FEATURE_OPT_FILTER", "FEATURE_GPIO", "FEATURE_FRAME_RATE", "FEATURE_ROI", "FEATURE_FLIP", "FEATURE_PIXEL_ADDRESSING", "FEATURE_PIXEL_FORMAT", "FEATURE_EXTENDED_SHUTTER", "FEATURE_AUTO_ROI", "FEATURE_LOOKUP_TABLE", "FEATURE_MEMORY_CHANNEL", "FEATURE_WHITE_SHADING", "FEATURE_ROTATE", "FEATURE_IMAGER_CLK_DIVISOR", "FEATURE_TRIG_WITH_CNTRLD_LIGHT", "FEATURE_MAX_PIXEL_SIZE"] ("uFeatureId IN")
            n123 = event-data() -> ("NewVal"=w365:dbl)  [unwired: 1 in, 4 out]
            n124 = To Double Precision Float(number=w365) -> (double precision float=w385:dbl)
            n125 = Build Array(w385) -> (w386:dbl[])
            n126 = call <vilib>:"MEPU-Acquisition-SetStreamState.vi"("hCamera IN"=w377, "uStreamState IN"=w381, "Error IN"=w376) -> ("hCamera OUT"=w383:u32, "Error OUT"=w382:errorcluster)  [unwired: 11 in]
            n127 = call <vilib>:"MEPU-CameraFeatures-SetFeature.vi"("hCamera IN"=w383, "uFeatureId IN"=w388, "uFlags IN"=w387, "pParms IN"=w386, "Error IN"=w382) -> ("hCamera OUT"=w370:u32, "Error OUT"=w384:errorcluster)  [unwired: 8 in, 1 out]
            n128 = case shown="Error" w384 {
              tunnel: [w399 errorcluster {"status"=FALSE, "code"=0, "source"=""} ("Error OUT")] -> w367
              tunnel: w384 -> [w399 _]
              frame No Error {
              }
              frame Error {
                n129 = One Button Dialog(message="Ocurrio un error con Gain") -> ()  [unwired: 1 in, 1 out]
              }
            }
            n130 = call <vilib>:"MEPU-CameraFeatures-GetFeature.vi"("hCamera IN"=w370, "uFeatureId IN"=w371, "Error IN"=w367) -> ("hCamera OUT"=w369:u32, "pParms OUT"=w372:dbl[], "Error OUT"=w368:errorcluster)  [unwired: 8 in, 2 out]
            n131 = Index Array(array=w372, index=0) -> (element=w364:dbl)
            n132 = property on="Gain" class="Slide (strict)"("Value"=w364) -> ()  [unwired: 2 in, 2 out]
            n133 = case shown="True" w375 {
              tunnel: w368 -> [w392 w397]
              tunnel: [w390 w396] -> w378
              tunnel: [w391 w395] -> w379
              tunnel: w369 -> [w389 w394]
              frame False {
                w393 = T9 2 items=["START_STREAM", "PAUSE_STREAM", "STOP_STREAM"] ("uStreamState IN")
                n134 = call <vilib>:"MEPU-Acquisition-SetStreamState.vi"("hCamera IN"=w389, "uStreamState IN"=w393, "Error IN"=w392) -> ("hCamera OUT"=w391:u32, "Error OUT"=w390:errorcluster)  [unwired: 11 in]
              }
              frame True {
                w398 = T9 0 items=["START_STREAM", "PAUSE_STREAM", "STOP_STREAM"] ("uStreamState IN")
                n135 = call <vilib>:"MEPU-Acquisition-SetStreamState.vi"("hCamera IN"=w394, "uStreamState IN"=w398, "Error IN"=w397) -> ("hCamera OUT"=w395:u32, "Error OUT"=w396:errorcluster)  [unwired: 11 in]
              }
            }
          }
        }
        n136 = call <vilib>:"Simple Error Handler.vi"("error in (no error)"=w77) -> ("error out"=w82:errorcluster)  [unwired: 1 in, 7 out]
        n137 = call <vilib>:"Simple Error Handler.vi"("error in (no error)"=w73) -> ("error out"=w72:errorcluster)  [unwired: 1 in, 7 out]
        n138 = case shown="Error" w82 {
          selector: w82 -> [w96 _]
          tunnel: [w96 errorcluster {"status"=FALSE, "code"=0, "source"=""} ("error IO")] -> w80
          tunnel: [FALSE ("T button?") w98] -> w81
          frame No Error {
          }
          frame Error {
            n139 = Two Button Dialog(message="An error was detected.\nDo you wish to continue execution?", 1:"Stop" ("F button name (\"Cancel\")"), 2:"Continue" ("T button name (\"OK\")")) -> (T button?=w99:bool)
            n140 = Not(x=w99) -> (.not. x?=w98:bool)
          }
        }
        n141 = case shown="Error" w72 {
          selector: w72 -> [w88 _]
          tunnel: [w88 errorcluster {"status"=FALSE, "code"=0, "source"=""} ("error IO")] -> w66
          tunnel: [FALSE ("T button?") w90] -> w67
          frame No Error {
          }
          frame Error {
            n142 = Two Button Dialog(message="An error was detected.\nDo you wish to continue execution?", 1:"Stop" ("F button name (\"Cancel\")"), 2:"Continue" ("T button name (\"OK\")")) -> (T button?=w91:bool)
            n143 = Not(x=w91) -> (.not. x?=w90:bool)
          }
        }
        n144 = property on="Stop App" class="Bool (strict)"() -> ("Value"=w71:bool)  [unwired: 2 in, 2 out]
        n145 = property on="Stop App" class="Bool (strict)"() -> ("Value"=w78:bool)  [unwired: 2 in, 2 out]
        n146 = Or(x=w67, y=w71) -> (x .or. y?=w69:bool)
        n147 = Or(x=w81, y=w78) -> (x .or. y?=w70:bool)
        n148 = Or(x=w70, y=w69) -> (x .or. y?=w68:bool)
      }
      n149 = call <vilib>:"Sound Output Clear.vi"("error in (no error)"=w12, "task ID"=w13) -> ()  [unwired: 9 in, 1 out]
      n150 = call <vilib>:"MEPU-Initialization-Uninitialize.vi"("hCamera IN"=w39, "Error IN"=w14) -> ()  [unwired: 13 in, 1 out]
    }
  }
